vi "Create Subpanel (by path).vi"(5 "Scrollbars (off)":T1, 7 "Sizing":T2, 8 "error in":errorcluster, 10 "Subpanel Ref":refnum<vi>, 11 "VI Path":path) -> (0 "error out":errorcluster, 3 "Philips Subpanel out":refnum<class "Flex UI Subpanel.lvclass">)   [LabVIEW 2014, in "Flex UI Subpanel.lvclass"]
uses:
  Flex UI Subpanel.lvclass
  Enum - Sizing.ctl
  Cluster - Scrollbar Visibility.ctl
  Flex UI (Parent)/Flex UI.lvclass
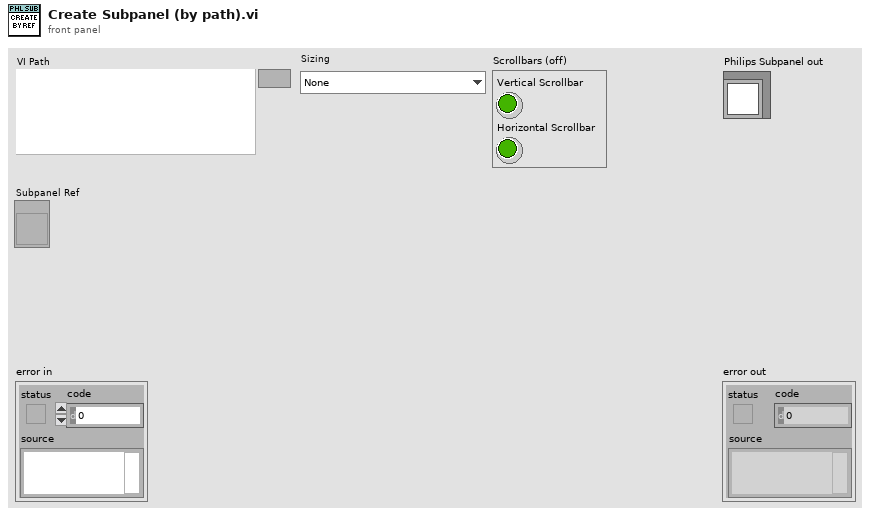
[diagram p1: front panel]
types:
  T1 = typedef "Flex UI Subpanel.lvclass/Cluster - Scrollbar Visibility.ctl" = cluster{"Vertical Scrollbar":bool, "Horizontal Scrollbar":bool}
  T2 = typedef "Flex UI Subpanel.lvclass/Enum - Sizing.ctl" = enum16{"None", "Largest Decoration", "Maximize"}
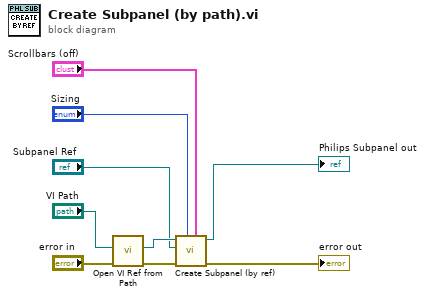
[diagram p0: block diagram]
diagram:
  n1 = call "Open VI Ref from Path.vi"("error in"="error in", "VI Path"="VI Path") -> ("error out"=w6:errorcluster, "VI Ref"=w4:refnum<vi>)  [unwired: 8 in]
  n2 = call "Create Subpanel (by ref).vi"("Scrollbars (off)"="Scrollbars (off)", "Sizing"="Sizing", "error in"=w6, "Subpanel Ref"="Subpanel Ref", "UI VI Reference (caller)"=w4) -> ("error out"=→"error out":errorcluster, "Philips Subpanel out"=→"Philips Subpanel out":refnum<class "Flex UI Subpanel.lvclass">)  [unwired: 5 in]
